vi "writeExpparams.vi"(8 "error in (no error)":errorcluster, 10 "示波器试验频率":dbl, 11 "试验时间":dbl) -> (0 "error out":errorcluster)   [LabVIEW 2014]
uses:
  <vilib>/addons/database/Connection.llb/DB Tools Open Connec (String).vi
  <vilib>/addons/database/Connection.llb/Conn Execute.vi
  <vilib>/addons/database/Recordset.llb/Rec Fetch Recordset Data (R).vi
  <vilib>/addons/database/Recordset.llb/Rec Destroy - Connection.vi
  <vilib>/addons/database/_DB Variant To Data/Database Variant To Data.xnode
  <vilib>/addons/database/NI_Database_API.lvlib
panel:
  out "连接的字符串":string
  out "余数":dbl
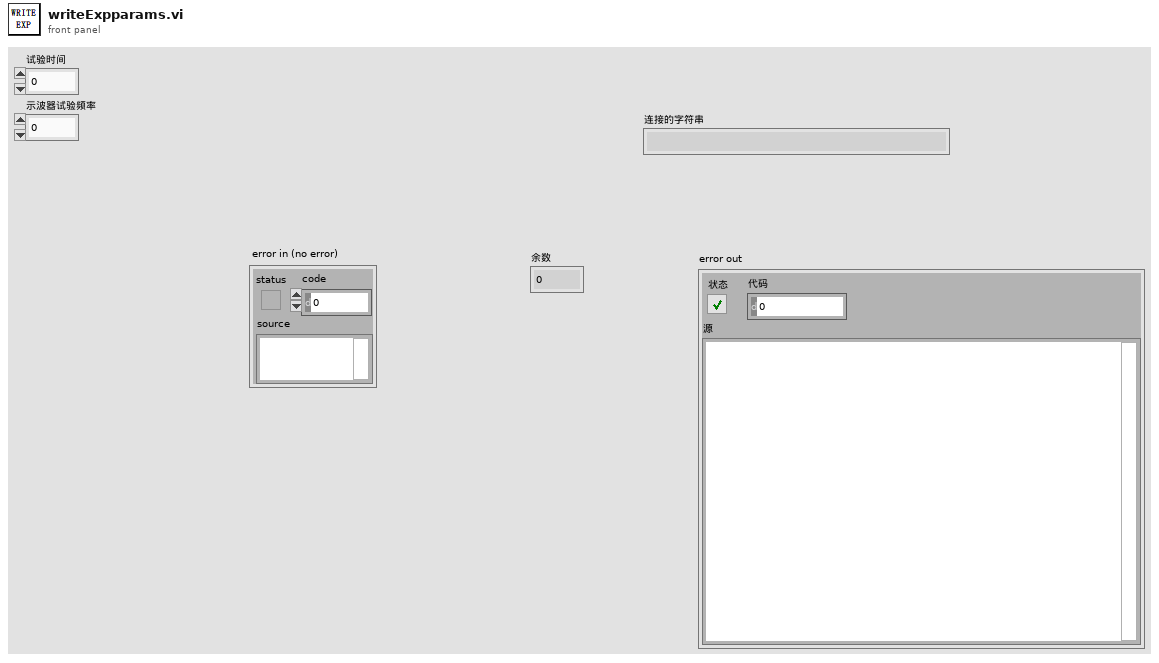
[diagram p1: front panel]
types:
  T1 = typedef "NI_Database_API.lvlib/Conn ObjectReference.ctl" = refnum<k1>
  T2 = typedef "NI_Database_API.lvlib/Rec ObjectReference.ctl" = refnum<k1>
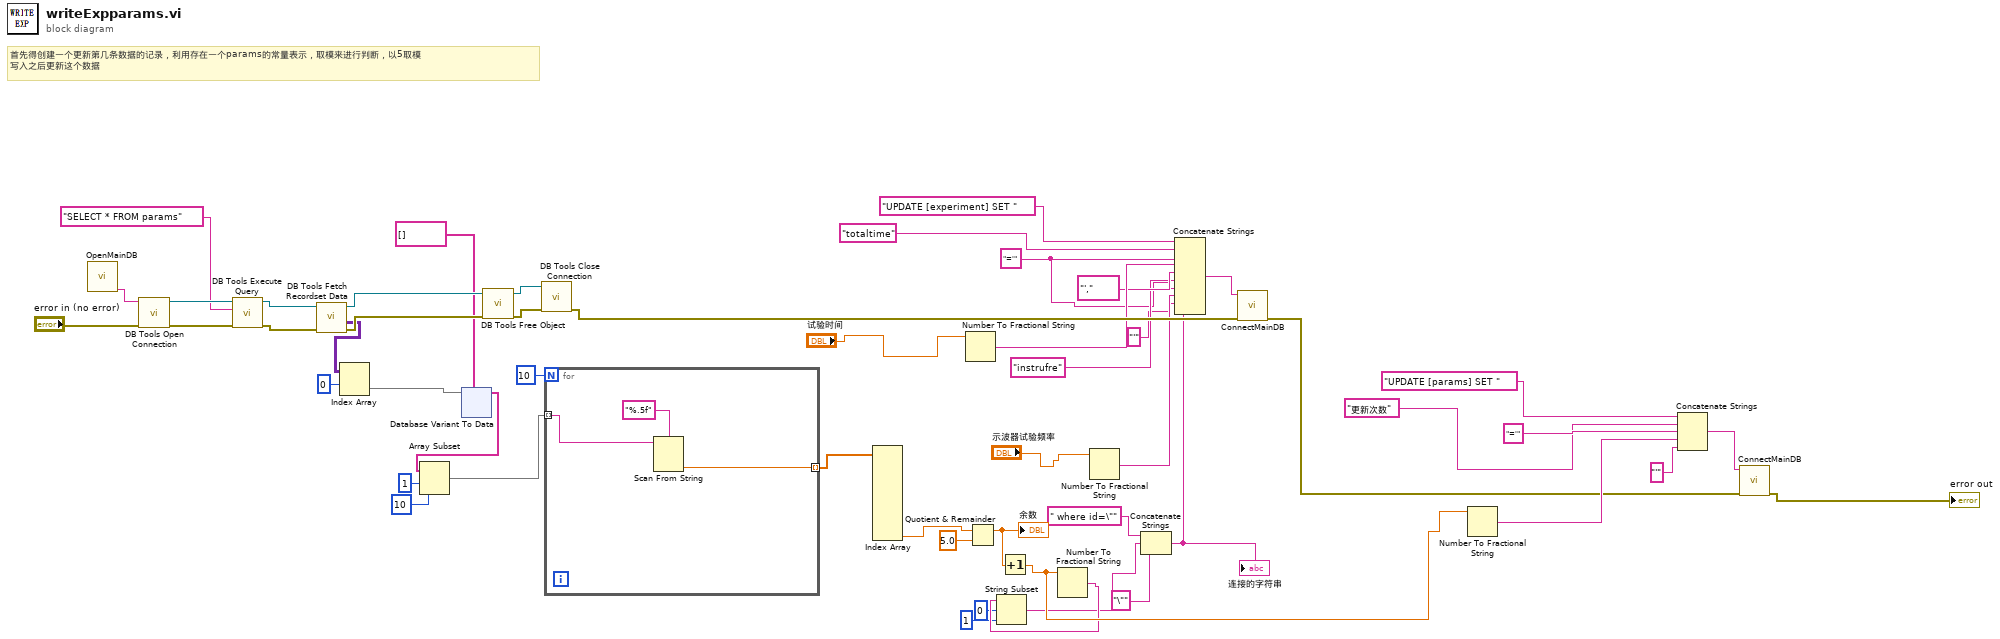
[diagram p0: block diagram]
diagram:
  w5 = "='"
  # "首先得创建一个更新第几条数据的记录，利用存在一个params的常量表示，取模来进行判断，以5取模\n写入之后更新这个数据"
  n1 = call "OpenMainDB.vi"() -> ("头信息"=w52:string)  [unwired: 11 in]
  n2 = call-poly <vilib>:"DB Tools Open Connection.vi"("error in (no error)"="error in (no error)", "connection information"=w52) -> ("error out"=w48:errorcluster, "connection reference"=w49:T1)  [unwired: 6 in]
  n3 = call-poly <vilib>:"DB Tools Execute Query.vi"("error in (no error)"=w48, "SQL query"="SELECT * FROM params", "connection reference"=w49) -> ("error out"=w47:errorcluster, "recordset reference"=w50:T2)  [unwired: 5 in]
  n4 = call-poly <vilib>:"DB Tools Fetch Recordset Data.vi"("error in (no error)"=w47, "recordset reference"=w50) -> ("error out"=w44:errorcluster, "recordset data"=w41:variant[][], "recordset reference out"=w45:T2)  [unwired: 3 in]
  n5 = Index Array(array=w41, index (row)=0 ("索引 (行)")) -> (element=w39:variant[])  [unwired: 1 in]
  n6 = xnode "Database Variant To Data"("database variant"=w39, "type"=string[] []) -> ("data"=w35:string[])  [unwired: 1 in, 1 out]
  n7 = Array Subset(array=w35, index=1 ("索引"), length=10 ("长度")) -> (w32:string[])
  n8 = call-poly <vilib>:"DB Tools Free Object.vi"("error in (no error)"=w44, "recordset reference"=w45) -> ("error out"=w42:errorcluster, "connection reference"=w43:T1)  [unwired: 8 in]
  n9 = call <vilib>:"DB Tools Close Connection.vi"("error in (no error)"=w42, "connection reference"=w43) -> ("error out"=w28:errorcluster)  [unwired: 5 in]
  n10 = for {
    N: 10 -> [_]
    tunnel: w32 -> [w55] mode=indexing
    tunnel: [w53] -> w36 mode=indexing
    n11 = Scan From String(format string="%.5f" ("格式字符串"), input string=w55) -> (output 1=w53:dbl)  [unwired: 3 in, 3 out]
  }
  n12 = Index Array(array=w36) -> (element #10=w30:dbl)  [unwired: 10 in, 9 out]
  n13 = Number To Fractional String(number="试验时间") -> (F-format string=w8:string)  [unwired: 3 in]
  n14 = Quotient & Remainder(x=w30, y=5.0) -> (x-y*floor(x/y)=w27:dbl)  [unwired: 1 out]
  "余数" <- w27
  n15 = Increment(x=w27) -> (x+1=w16:dbl)
  n16 = Number To Fractional String(number=w16) -> (F-format string=w15:string)  [unwired: 3 in]
  n17 = String Subset(string=w15, offset (0)=0 ("偏移量(0)"), length (rest)=1 ("长度（剩余）")) -> (substring=w13:string)
  n18 = Number To Fractional String(number="示波器试验频率") -> (F-format string=w4:string)  [unwired: 3 in]
  n19 = Concatenate Strings(" where id=\"" ("多行字符串"), w13, "\"") -> (w1:string)
  "连接的字符串" <- w1
  n20 = Concatenate Strings("UPDATE [experiment] SET ", "totaltime" ("多行字符串"), w5, w8, "',", "instrufre" ("多行字符串"), w5, w4, "'", w1) -> (w29:string)
  n21 = call "ConnectMainDB.vi"("error in (no error)"=w28, "SQL query"=w29) -> ("error out"=w17:errorcluster)  [unwired: 8 in, 1 out]
  n22 = Number To Fractional String(number=w16) -> (F-format string=w24:string)  [unwired: 3 in]
  n23 = Concatenate Strings("UPDATE [params] SET ", "更新次数" ("多行字符串"), "='", w24, "'") -> (w19:string)
  n24 = call "ConnectMainDB.vi"("error in (no error)"=w17, "SQL query"=w19) -> ("error out"=→"error out":errorcluster)  [unwired: 8 in, 1 out]
